vi "Load Trigger Model ExternalTrigger Template.vi"(0 "VISA resource name":refnum<visa-resource-name>, 1 "Delay":dbl, 2 "Reading Block":u16(ring) items=["Active", "Measure", "Digitize"], 5 "Digital In Line":u32=1 min=1 max=7 step=1, 7 "Digital Out Line":u32=1 min=1 max=6 step=1, 9 "Count":i16, 11 "error in (no error)":errorcluster, 12 "Reading Buffer":string="defbuffer1") -> (4 "VISA resource name out":refnum<visa-resource-name>, 15 "error Out (no error)":errorcluster)   [LabVIEW 2018, in "Keithley DMM7512.lvlib"]
doc: "This VI loads a predefined trigger model configuration that sets up an external trigger through the digital I/O."
uses:
  <instrlib>/Keithley DMM7512/Keithley DMM7512.lvlib
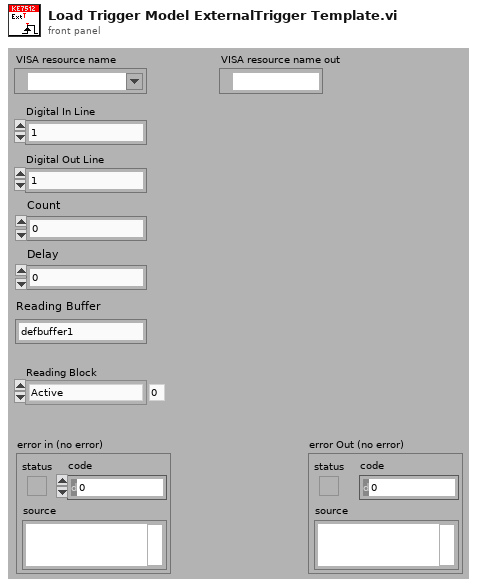
[diagram p1: front panel]
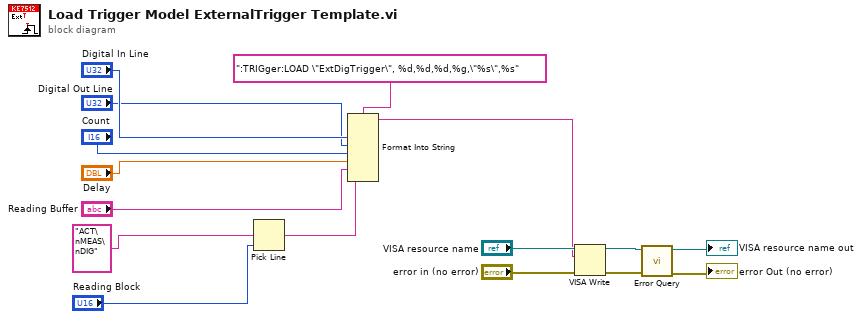
[diagram p0: block diagram]
diagram:
  n1 = Pick Line(multi-line string="ACT\nMEAS\nDIG", line index="Reading Block") -> (output string=w1:string)  [unwired: 1 in]
  n2 = Format Into String(format string=":TRIGger:LOAD \"ExtDigTrigger\", %d,%d,%d,%g,\"%s\",%s", "Digital In Line", "Digital Out Line", "Count", "Delay", "Reading Buffer", w1) -> (resulting string=w13:string)  [unwired: 2 in, 1 out]
  n3 = VISA Write(VISA resource name="VISA resource name", write buffer=w13, error in (no error)="error in (no error)") -> (VISA resource name out=w12:refnum<visa-resource-name>, error out=w10:errorcluster)  [unwired: 1 out]
  n4 = call <instrlib>:"Error Query.vi"("error in (no error)"=w10, "VISA resource name"=w12) -> ("error out"=→"error Out (no error)":errorcluster, "VISA resource name out"=→"VISA resource name out":refnum<visa-resource-name>)  [unwired: 6 in, 2 out]
